vi "M2p_AD_Std.vi"() -> ()   [LabVIEW 2015]
uses:
  spcm_library/spcm_gui_common.llb/element_mode.ctl
  spcm_library/spcm_gui_m2p.llb/element_m2p_ai_channel.ctl
  spcm_library/spcm_gui_m2p.llb/element_m2p_ai_trigger.ctl
  spcm_library/spcm_gui_m2p.llb/element_m2p_clock.ctl
  spcm_library/spcm_gui_common.llb/element_device.ctl
  spcm_library/spcm_gui_common.llb/element_device_infos.ctl
  spcm_library/spcm_gui_m2p.llb/element_m2p_ai_multi_purpose_io.ctl
panel:
  in  "Multi Purpose IO Lines":T1={"X0 Mode"=0, "X1 Mode"=0, "X2 Mode"=0, "X3 Mode"=0, "X0 ASync Send Pulse"=FALSE, "X1 ASync Send Pulse"=FALSE, "X2 ASync Send Pulse"=FALSE, "X3 ASync Send Pulse"=FALSE, "X1 Trigger Mode"=0, "X2 Trigger Mode"=0, "X3 Trigger Mode"=0, "X1 Pulsewidth"=0, "X2 Pulsewidth"=0, "X3 Pulsewidth"=0, "ASync Read Button"=FALSE, "ASync Read"=0, "AI"=TRUE} {"X3 Mode" items=["Disable", "Asynchronous Out", "Asynchronous In", "Trigger Out", "Trigger In", "Clock Out", "Digital In", "Show Run State", "Show Arm State", "Show Sync Arm State"]; "X2 Mode" items=["Disable", "Asynchronous Out", "Asynchronous In", "Trigger Out", "Trigger In", "Clock Out", "Digital In", "Show Run State", "Show Arm State", "Show Sync Arm State"]; "X3 Trigger Mode" items=["Pos. Edge", "Neg. Edge", "Any Edge", "High Level", "Low Level", "PW Long Pos.", "PW Long Neg.", "PW Short Pos.", "PW Short Neg."]; "X2 Trigger Mode" items=["Pos. Edge", "Neg. Edge", "Any Edge", "High Level", "Low Level", "PW Long Pos.", "PW Long Neg.", "PW Short Pos.", "PW Short Neg."]; "X1 Trigger Mode" items=["Pos. Edge", "Neg. Edge", "Any Edge", "High Level", "Low Level", "PW Long Pos.", "PW Long Neg.", "PW Short Pos.", "PW Short Neg."]; "X1 Mode" items=["Disable", "Asynchronous Out", "Asynchronous In", "Trigger Out", "Trigger In", "Clock Out", "Digital In", "Show Run State", "Show Arm State", "Show Sync Arm State"]; "X0 Mode" items=["Disable", "Asynchronous Out", "Trigger Out", "Clock Out", "Show Run State", "Show Arm State", "Show Sync Arm State"]}
  out "Device Infos":T2={"Device Name"="M4i.4451-Exp", "Serial Number"=1122.0, "Mem (MB)"=4096.0}
  in  "Device":T3 {"Device" items=["Card", "digitizerNETBOX"]}
  in  "Clock Settings":T4={"Clock Mode"=0, "Sampling Rate (kHz)"=10000.0, "Clock Output"=FALSE, "Termination"=FALSE, "Ref. Clock (MHz)"=10.0, "Threshold (mV)"=1500} {"Threshold (mV)" min=-5000 max=5000; "Clock Mode" items=["Internal Clock Quartz", "External Clock", "External Reference Clock"]; "Ref. Clock (MHz)" min=0.0 max=125000.0; "Sampling Rate (kHz)" min=1.0 max=5000000.0}
  in  "Trigger Settings":T5={"Trigger Source"=0, "External Trigger"=0, "Level 0 Ext"=1500, "Ext Trig Term"=FALSE, "Channel Trigger"=0, "Level 0 Ch"=0, "Level 1 Ch"=0, "Trigger Delay (Samples)"=0} {"Channel Trigger" items=["None", "Pos. Edge", "Neg. Edge", "Any Edge", "Pos. Rearm", "Neg. Rearm", "Enter Window", "Leave Window", "In Win", "Out Win"]; "External Trigger" items=["None", "Pos. Edge", "Neg. Edge", "Any Edge", "High Level", "Low Level"]; "Trigger Source" items=["Software Trigger", "External Trigger", "Channel 0 Trigger", "Channel 1 Trigger", "Channel 2 Trigger", "Channel 3 Trigger", "Channel 4 Trigger", "Channel 5 Trigger", "Channel 6 Trigger", "Channel 7 Trigger"]; "Trigger Delay (Samples)" max=65535 step=1}
  in  "Quit Button":bool
  in  "AI Channel 7":T6={"Enable"=TRUE, "Input Range "=2, "Termination"=0, "Input Type"=0, "Offset"=0} {"Input Type" items=["Single-ended", "Differential"]; "Termination" items=["1 MOhm", "50 Ohm"]; "Input Range" items=["±200 mV", "±500 mV", "±1000 mV", "±2000 mV", "±5000 mV", "±10000 mV"]}
  in  "AI Channel 6":T6={"Enable"=TRUE, "Input Range "=2, "Termination"=0, "Input Type"=0, "Offset"=0} {"Input Type" items=["Single-ended", "Differential"]; "Termination" items=["1 MOhm", "50 Ohm"]; "Input Range" items=["±200 mV", "±500 mV", "±1000 mV", "±2000 mV", "±5000 mV", "±10000 mV"]}
  in  "AI Channel 5":T6={"Enable"=TRUE, "Input Range "=2, "Termination"=0, "Input Type"=0, "Offset"=0} {"Input Type" items=["Single-ended", "Differential"]; "Termination" items=["1 MOhm", "50 Ohm"]; "Input Range" items=["±200 mV", "±500 mV", "±1000 mV", "±2000 mV", "±5000 mV", "±10000 mV"]}
  in  "AI Channel 4":T6={"Enable"=TRUE, "Input Range "=2, "Termination"=0, "Input Type"=0, "Offset"=0} {"Input Type" items=["Single-ended", "Differential"]; "Termination" items=["1 MOhm", "50 Ohm"]; "Input Range" items=["±200 mV", "±500 mV", "±1000 mV", "±2000 mV", "±5000 mV", "±10000 mV"]}
  in  "AI Channel 3":T6={"Enable"=TRUE, "Input Range "=2, "Termination"=0, "Input Type"=0, "Offset"=0} {"Input Type" items=["Single-ended", "Differential"]; "Termination" items=["1 MOhm", "50 Ohm"]; "Input Range" items=["±200 mV", "±500 mV", "±1000 mV", "±2000 mV", "±5000 mV", "±10000 mV"]}
  in  "AI Channel 2":T6={"Enable"=TRUE, "Input Range "=2, "Termination"=0, "Input Type"=0, "Offset"=0} {"Input Type" items=["Single-ended", "Differential"]; "Termination" items=["1 MOhm", "50 Ohm"]; "Input Range" items=["±200 mV", "±500 mV", "±1000 mV", "±2000 mV", "±5000 mV", "±10000 mV"]}
  in  "AI Channel 1":T6={"Enable"=TRUE, "Input Range "=2, "Termination"=0, "Input Type"=0, "Offset"=0} {"Input Type" items=["Single-ended", "Differential"]; "Termination" items=["1 MOhm", "50 Ohm"]; "Input Range" items=["±200 mV", "±500 mV", "±1000 mV", "±2000 mV", "±5000 mV", "±10000 mV"]}
  in  "AI Channel 0":T6={"Enable"=TRUE, "Input Range "=2, "Termination"=0, "Input Type"=0, "Offset"=0} {"Input Type" items=["Single-ended", "Differential"]; "Termination" items=["1 MOhm", "50 Ohm"]; "Input Range" items=["±200 mV", "±500 mV", "±1000 mV", "±2000 mV", "±5000 mV", "±10000 mV"]}
  in  "Loop Button":bool
  in  "Singleshot Button":bool
  out "Write Setup":bool
  out "Status":string
  in  "Force Trigger Button":bool
  in  "Stop Button":bool
  out "Display Data":sgl[][](graph)
  in  "Mode Setup":T7={"Mode"=0, "Mem"=16384, "Seg"=1024, "Post"=8192, "Pre"=32, "ABA"=16} {"Mode" items=["Singleshot", "Multiple Recording", "Gated Sampling", "ABA Mode"]; "ABA" min=2 max=65535 step=1; "Post" min=4 step=4; "Mem" min=8 step=4; "Pre" min=4 max=8176 step=4; "Seg" min=8 step=4}
  # "M2p AD Standard Example"
  # "Range"
  # "Term"
  # "Type"
  # "Offset"
  # "Mode Settings"
  # "Trigger Settings"
  # "Ch0"
  # "Ch1"
  # "Ch2"
  # "Clock Settings"
  # "Ch3"
  # "Ch4"
  # "Ch5"
  # "Ch6"
  # "Multi Purpose IO"
  # "Ch7"
  # "Mode"
  # "ASync Write"
  # "Trig-Mode"
  # "Trig-Pulsewidth"
  # "ASync Read"
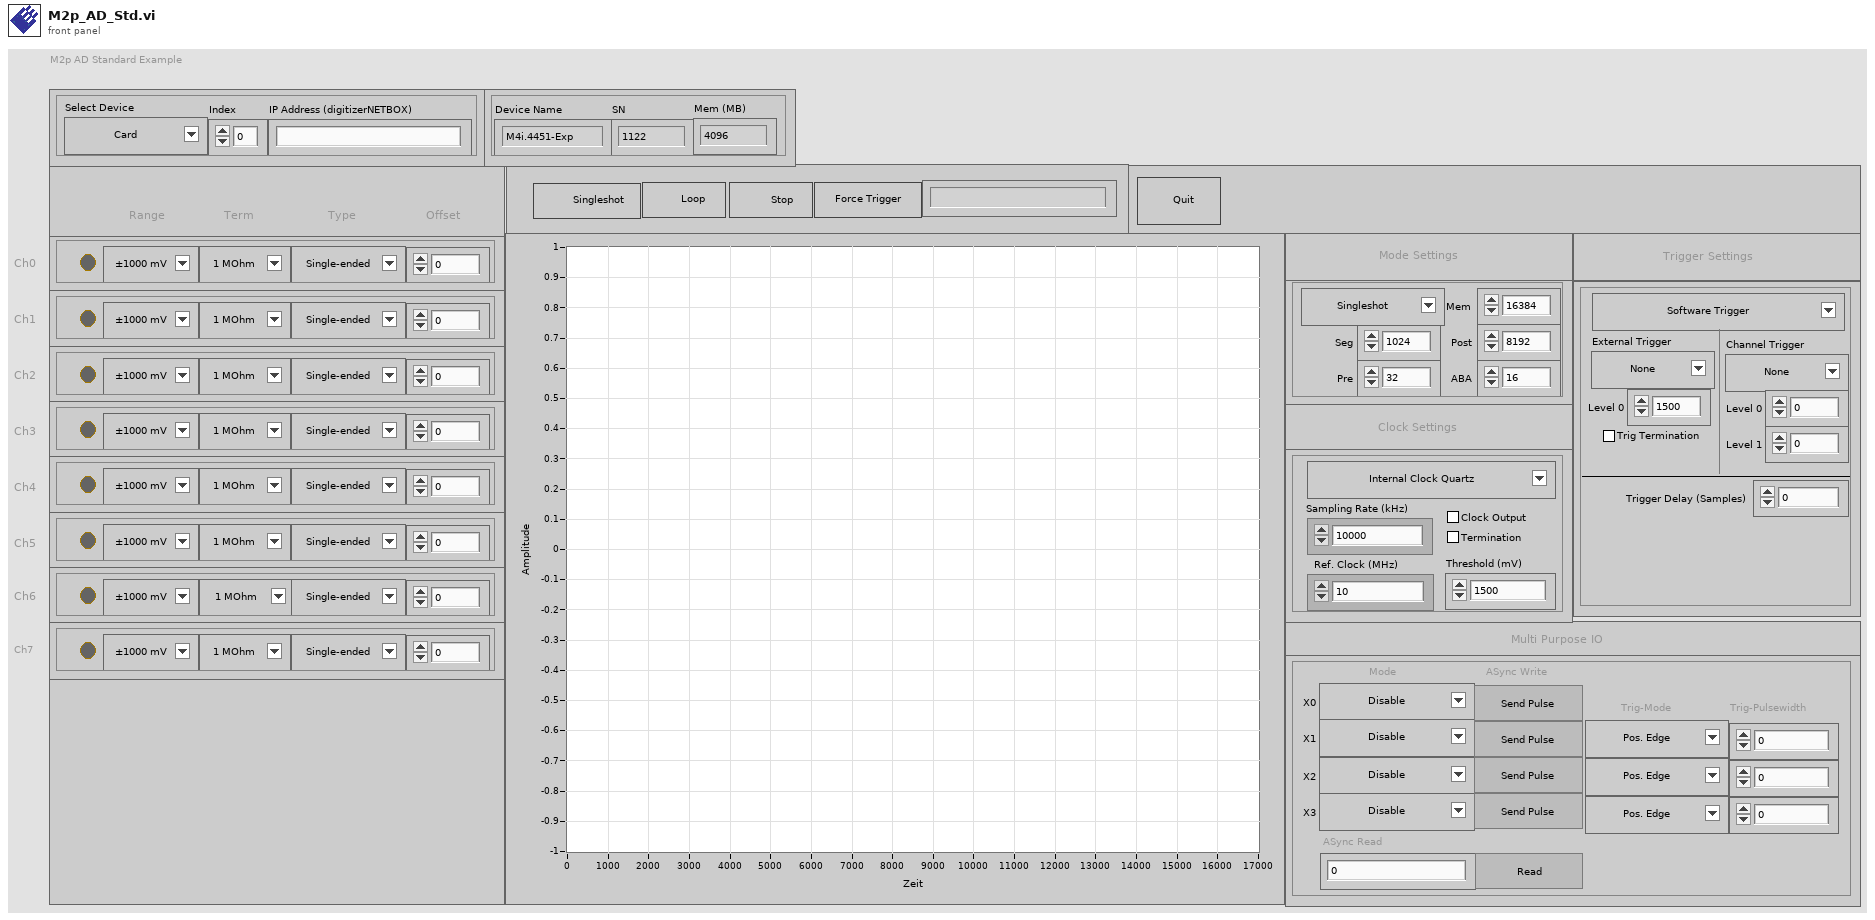
[diagram p1: front panel]
types:
  T1 = typedef "element_m2p_ai_multi_purpose_io.ctl" = cluster{"X0 Mode":u16, "X1 Mode":u16, "X2 Mode":u16, "X3 Mode":u16, "X0 ASync Send Pulse":bool, "X1 ASync Send Pulse":bool, "X2 ASync Send Pulse":bool, "X3 ASync Send Pulse":bool, "X1 Trigger Mode":u16, "X2 Trigger Mode":u16, "X3 Trigger Mode":u16, "X1 Pulsewidth":u32, "X2 Pulsewidth":u32, "X3 Pulsewidth":u32, "ASync Read Button":bool, "ASync Read":i32, "AI":bool}
  T2 = typedef "element_device_infos.ctl" = cluster{"Device Name":string, "Serial Number":dbl, "Mem (MB)":dbl}
  T3 = typedef "element_device.ctl" = cluster{"Index":dbl, "IP Address":string, "Device":u16}
  T4 = typedef "element_m2p_clock.ctl" = cluster{"Clock Mode":u16, "Sampling Rate (kHz)":dbl, "Clock Output":bool, "Termination":bool, "Ref. Clock (MHz)":dbl, "Threshold (mV)":i32}
  T5 = typedef "element_m2p_ai_trigger.ctl" = cluster{"Trigger Source":u16, "External Trigger":u16, "Level 0 Ext":i32, "Ext Trig Term":bool, "Channel Trigger":u16, "Level 0 Ch":i32, "Level 1 Ch":i32, "Trigger Delay (Samples)":u32}
  T6 = typedef "element_m2p_ai_channel.ctl" = cluster{"Enable":bool, "Input Range ":u16, "Termination":u16, "Input Type":u16, "Offset":i32}
  T7 = typedef "element_mode.ctl" = cluster{"Mode":u16, "Mem":u32, "Seg":u32, "Post":u32, "Pre":u32, "ABA":u32}
  T8 = enum16{"Idle", "Init", "Write Setup", "Start", "Acquire", "Read Data", "Stop", "Quit"}
  T9 = cluster{"Card Type":i32, "Inst Mem (high part)":i32, "Inst Mem (low part)":i32, "Serial Number":i32, "Function Type":i32, "Installed Features":i32, "Base Card Version":i32, "Module Version":i32, "Extension Version":i32, "Production Date":i32, "Max Sampling Rate":i32, "Max Channels":i32, "Demo Card":i32}
  T10 = cluster{"Card Name":string, "SN":i32, "Mem (MB)":i32}
  T11 = cluster{"AI Channels":i32, "AI Ranges":i32, "Input Ranges (mV)":i32[], "Programmable Offset":i32, "Termination Available":bool, "SE/Diff switchable":bool, "Offset in per cent/mV":bool, "Offset Calibration":bool, "Gain Calibration":bool, "Offset with open inputs":bool, "AI Range Strings[]":string[], "Bit Resolution":i32, "AC Coupling available":bool, "BW Limit available":bool, "AI Path count":i32}
  T12 = enum16{"Idle", "Init", "Write Setup", "Start", "Acquire", "Read Data", "Quit"}
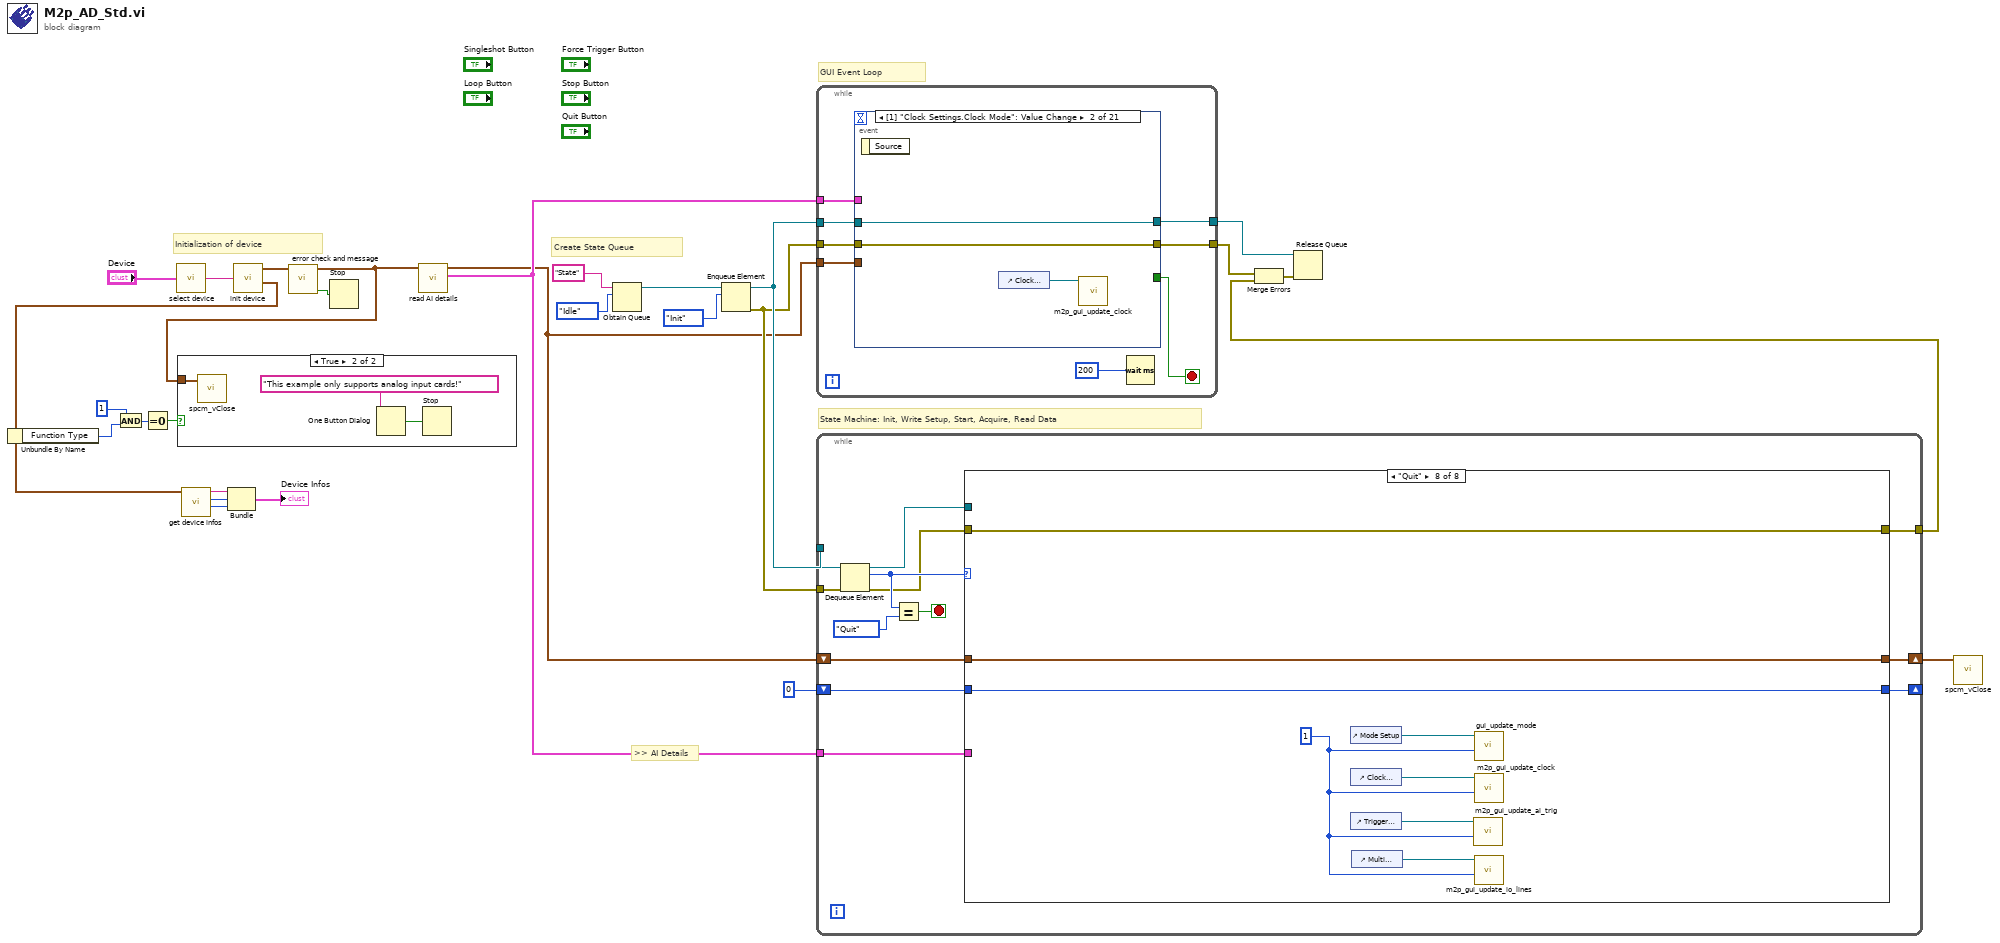
[diagram p0: block diagram]
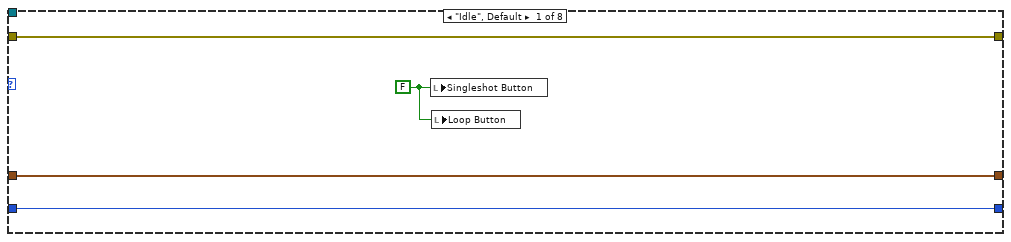
[diagram p3: hidden frame]
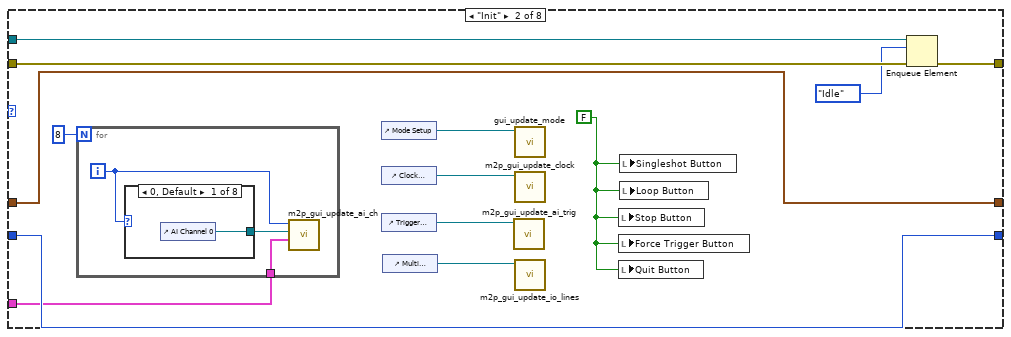
[diagram p4: hidden frame]
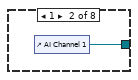
[diagram p5: hidden frame]
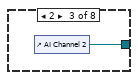
[diagram p6: hidden frame]
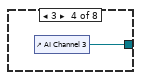
[diagram p7: hidden frame]
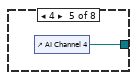
[diagram p8: hidden frame]
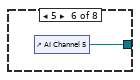
[diagram p9: hidden frame]
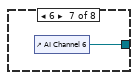
[diagram p10: hidden frame]
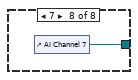
[diagram p11: hidden frame]
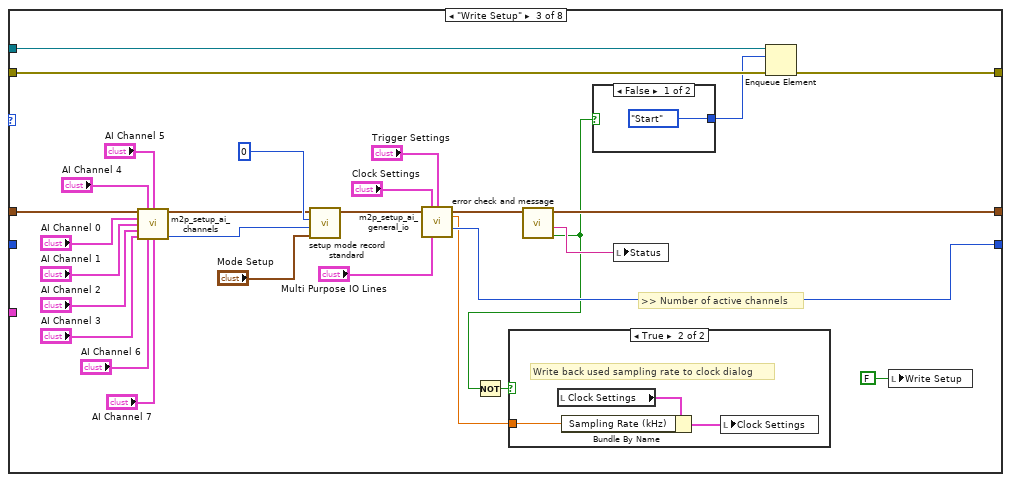
[diagram p12: hidden frame]
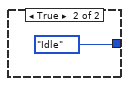
[diagram p14: hidden frame]
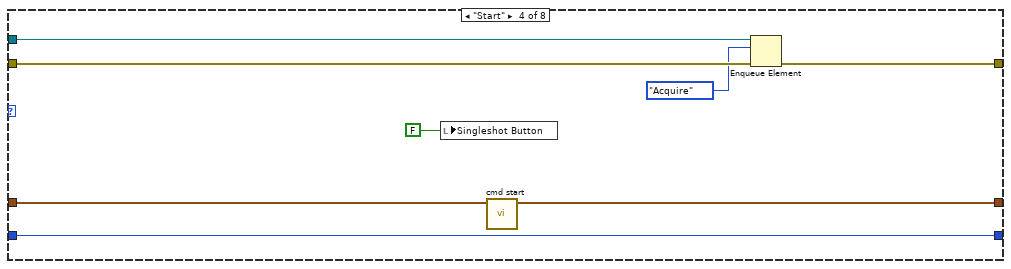
[diagram p15: hidden frame]
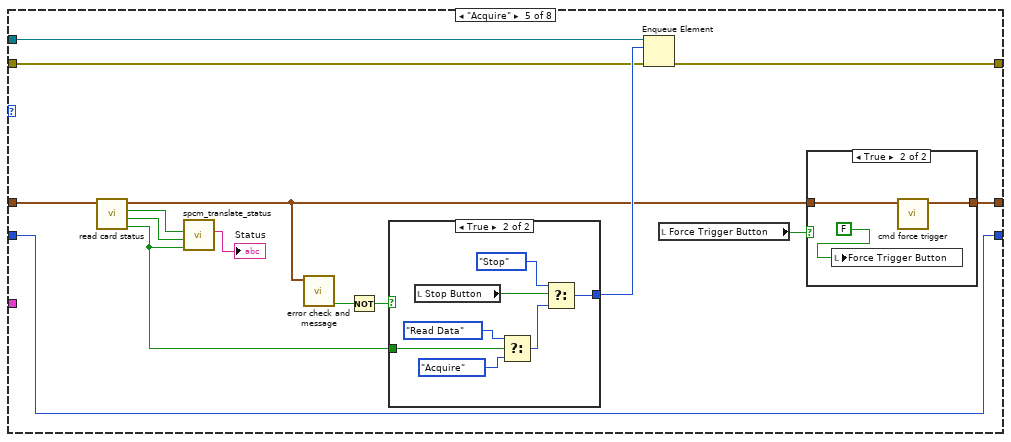
[diagram p16: hidden frame]
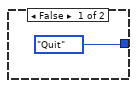
[diagram p17: hidden frame]
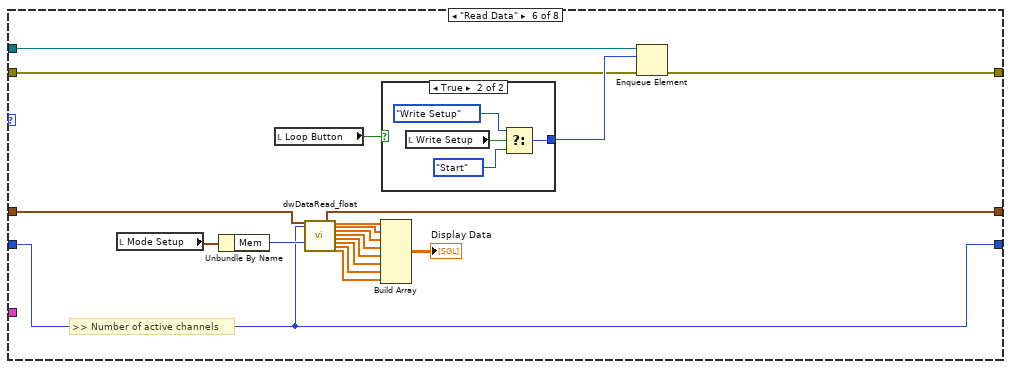
[diagram p19: hidden frame]
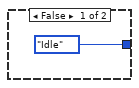
[diagram p20: hidden frame]
diagram:
  # ">> AI Details"
  # "Initialization of device"
  # "Create State Queue"
  # "State Machine: Init, Write Setup, Start, Acquire, Read Data"
  # "GUI Event Loop"
  n1 = call "select device.vi"("Device"="Device") -> ("device string"=w28:string)  [unwired: 4 in]
  n2 = call "init device.vi"("Device String"=w28) -> ("Card Info Out"=w27:cluster{"Card Handle":u64, "Error Code":u32}, "Card Information"=w13:T9)  [unwired: 4 in]
  n3 = Unbundle By Name(w13) -> ("Function Type"=w17:i32)
  n4 = And(x=1, y=w17) -> (x .and. y?=w16:i32)
  n5 = Equal To 0?(x=w16) -> (x = 0?=w14:bool)
  n6 = call "get device infos.vi"("Card Information"=w13) -> ("Mem (MB)"=w20:i32, "SN"=w19:i32, "Card Name"=w18:string)  [unwired: 8 in]
  n7 = Bundle("Card Name"=w18, "SN"=w19, "Mem (MB)"=w20) -> (→"Device Infos":T10)  [unwired: 1 in]
  n8 = call "error check and message.vi"("Card Info In"=w27) -> ("Error occurred"=w26:bool, "Card Info Out"=w5:cluster{"Card Handle":u64, "Error Code":u32})  [unwired: 4 in, 1 out]
  n9 = case shown="True" w14 {
    tunnel: w5 -> [_ w29]
    frame False {
    }
    frame True {
      n10 = call "spcm_vClose.vi"("Card Info In"=w29) -> ()  [unwired: 7 in]
      n11 = One Button Dialog(message="This example only supports analog input cards!") -> (true=w30:bool)  [unwired: 1 in]
      n12 = Stop(stop? (T)=w30) -> ()
    }
  }
  n13 = Stop(stop? (T)=w26) -> ()
  n14 = call "read AI details.vi"("Card Info In"=w5) -> ("AI Details"=w4:T11, "Card Info Out"=w3:cluster{"Card Handle":u64, "Error Code":u32})  [unwired: 5 in]
  n15 = Obtain Queue(name (unnamed)="State", element data type=T8."Idle") -> (queue out=w23:refnum<queue>)  [unwired: 3 in, 2 out]
  n16 = Enqueue Element(queue=w23, element=T8."Init") -> (queue out=w24:refnum<queue>, error out=w8:errorcluster)  [unwired: 2 in, 1 out]
  n17 = while {
    tunnel: w24 -> [w37]
    tunnel: [w38] -> w9
    tunnel: [w34] -> w12
    tunnel: w8 -> [w35]
    tunnel: w4 -> [w33]
    tunnel: w3 -> [w32]
    stop <- w36 stop-if-true
    n18 = event shown="[1] \"Clock Settings.Clock Mode\": Value Change" {
      selector: _ -> [_ _ _ _ _ _ _ _ _ _ _ _ _ _ _ _ _ _ _ _ _]
      dyn-events: _ -> [_ _ _ _ _ _ _ _ _ _ _ _ _ _ _ _ _ _ _ _ _]
      timeout: _ -> [_ _ _ _ _ _ _ _ _ _ _ _ _ _ _ _ _ _ _ _ _]
      tunnel: [_ _ _ _ _ _ _ _ _ _ _ _ _ _ _ _ _ _ _ TRUE _] -> w36
      tunnel: [w41 w45 w48 w50 w58 w63 w68 w73 w79 w84 w89 w94 w99 w104 w109 w114 w119 w124 w129 w134 w138] -> w38
      tunnel: w37 -> [w41 w45 w48 w50 w58 w63 w68 w73 w79 w84 w89 w94 w99 w104 w109 w114 w119 w123 w128 w135 w138]
      tunnel: [w40 w44 w47 w51 w57 w62 w67 w72 w78 w83 w88 w93 w98 w103 w108 w113 w118 w121 w126 w132 w137] -> w34
      tunnel: w35 -> [w40 w44 w47 w51 w57 w62 w67 w72 w78 w83 w88 w93 w98 w103 w108 w113 w118 w122 w127 w131 w137]
      tunnel: w33 -> [_ _ _ _ _ _ _ _ _ w80 w86 w91 w96 w101 w106 w111 w116 _ _ _ _]
      tunnel: w32 -> [_ _ _ w53 w55 w60 w65 w70 w77 _ _ _ _ _ _ _ _ _ _ _ _]
      event Value Change {
        n19 = event-data ("Ereignisdatenknoten")() -> ()  [unwired: 1 in, 1 out]
        n20 = control-ref of="Mode Setup"() -> (w42:refnum<vi>)
        n21 = call "gui_update_mode.vi"("Referenz Mode Settings"=w42) -> ()  [unwired: 11 in]
      }
      event Value Change {
        n22 = event-data() -> ()  [unwired: 1 in, 1 out]
        n23 = control-ref of="Clock Settings"() -> (w43:refnum<vi>)
        n24 = call "m2p_gui_update_clock.vi"("Cluster Reference"=w43) -> ()  [unwired: 11 in]
      }
      event Value Change {
        n25 = event-data() -> ()  [unwired: 1 in, 1 out]
        n26 = control-ref of="Trigger Settings"() -> (w46:refnum<vi>)
        n27 = call "m2p_gui_update_ai_trig.vi"("Trigger Settings Reference"=w46) -> ()  [unwired: 10 in]
      }
      event Value Change {
        n28 = event-data() -> ()  [unwired: 1 in, 1 out]
        n29 = local read "Multi Purpose IO Lines"() -> (w52:T1)
        n30 = control-ref of="Multi Purpose IO Lines"() -> (w49:refnum<vi>)
        n31 = call "m2p_gui_update_io_lines.vi"("Cluster Reference"=w49) -> ()  [unwired: 11 in]
        n32 = call "setup M2p IO lines.vi"("Multi Purpose IO Lines"=w52, "Card Info In"=w53) -> ()  [unwired: 1 in, 1 out]
      }
      event Value Change {
        n33 = event-data() -> ()  [unwired: 1 in, 1 out]
        n34 = call "write M2p async io.vi"("Card Info In"=w55, "XIO Index"=0) -> ()  [unwired: 4 in, 1 out]
        n35 = One Button Dialog(message="X0: Send Pulse") -> ()  [unwired: 1 in, 1 out]
      }
      event Value Change {
        n36 = event-data() -> ()  [unwired: 1 in, 1 out]
        n37 = call "write M2p async io.vi"("Card Info In"=w60, "XIO Index"=1) -> ()  [unwired: 4 in, 1 out]
        n38 = One Button Dialog(message="X1: Send Pulse") -> ()  [unwired: 1 in, 1 out]
      }
      event Value Change {
        n39 = event-data() -> ()  [unwired: 1 in, 1 out]
        n40 = call "write M2p async io.vi"("Card Info In"=w65, "XIO Index"=2) -> ()  [unwired: 4 in, 1 out]
        n41 = One Button Dialog(message="X2: Send Pulse") -> ()  [unwired: 1 in, 1 out]
      }
      event Value Change {
        n42 = event-data() -> ()  [unwired: 1 in, 1 out]
        n43 = call "write M2p async io.vi"("Card Info In"=w70, "XIO Index"=3) -> ()  [unwired: 4 in, 1 out]
        n44 = One Button Dialog(message="X3: Send Pulse") -> ()  [unwired: 1 in, 1 out]
      }
      event Value Change {
        n45 = event-data() -> ()  [unwired: 1 in, 1 out]
        n46 = call "read M2p async io.vi"("Card Info In"=w77) -> ("ASync Read"=w76:i32)  [unwired: 5 in, 1 out]
        n47 = local read "Multi Purpose IO Lines"() -> (w75:T1)
        n48 = Bundle By Name(cluster=w75, "ASync Read"=w76) -> (w74:T1)
        n49 = local write "Multi Purpose IO Lines"(w74) -> ()
      }
      event Value Change {
        n50 = event-data() -> ()  [unwired: 1 in, 1 out]
        n51 = control-ref of="AI Channel 0"() -> (w81:refnum<vi>)
        n52 = call "m2p_gui_update_ai_ch.vi"("AI Details"=w80, "Cluster Referenz"=w81, "Channel Index"=0) -> ()  [unwired: 9 in]
      }
      event Value Change {
        n53 = event-data() -> ()  [unwired: 1 in, 1 out]
        n54 = control-ref of="AI Channel 1"() -> (w85:refnum<vi>)
        n55 = call "m2p_gui_update_ai_ch.vi"("AI Details"=w86, "Cluster Referenz"=w85, "Channel Index"=1) -> ()  [unwired: 9 in]
      }
      event Value Change {
        n56 = event-data() -> ()  [unwired: 1 in, 1 out]
        n57 = control-ref of="AI Channel 2"() -> (w90:refnum<vi>)
        n58 = call "m2p_gui_update_ai_ch.vi"("AI Details"=w91, "Cluster Referenz"=w90, "Channel Index"=2) -> ()  [unwired: 9 in]
      }
      event Value Change {
        n59 = event-data() -> ()  [unwired: 1 in, 1 out]
        n60 = control-ref of="AI Channel 3"() -> (w95:refnum<vi>)
        n61 = call "m2p_gui_update_ai_ch.vi"("AI Details"=w96, "Cluster Referenz"=w95, "Channel Index"=3) -> ()  [unwired: 9 in]
      }
      event Value Change {
        n62 = event-data() -> ()  [unwired: 1 in, 1 out]
        n63 = control-ref of="AI Channel 4"() -> (w100:refnum<vi>)
        n64 = call "m2p_gui_update_ai_ch.vi"("AI Details"=w101, "Cluster Referenz"=w100, "Channel Index"=4) -> ()  [unwired: 9 in]
      }
      event Value Change {
        n65 = event-data() -> ()  [unwired: 1 in, 1 out]
        n66 = control-ref of="AI Channel 5"() -> (w105:refnum<vi>)
        n67 = call "m2p_gui_update_ai_ch.vi"("AI Details"=w106, "Cluster Referenz"=w105, "Channel Index"=5) -> ()  [unwired: 9 in]
      }
      event Value Change {
        n68 = event-data() -> ()  [unwired: 1 in, 1 out]
        n69 = control-ref of="AI Channel 6"() -> (w110:refnum<vi>)
        n70 = call "m2p_gui_update_ai_ch.vi"("AI Details"=w111, "Cluster Referenz"=w110, "Channel Index"=6) -> ()  [unwired: 9 in]
      }
      event Value Change {
        n71 = event-data() -> ()  [unwired: 1 in, 1 out]
        n72 = control-ref of="AI Channel 7"() -> (w115:refnum<vi>)
        n73 = call "m2p_gui_update_ai_ch.vi"("AI Details"=w116, "Cluster Referenz"=w115, "Channel Index"=7) -> ()  [unwired: 9 in]
      }
      event "Singleshot Button", "Loop Button": Value Change {
        n74 = event-data() -> ()  [unwired: 1 in, 1 out]
        n75 = Enqueue Element(queue=w123, element=T8."Write Setup", error in (no error)=w122) -> (queue out=w124:refnum<queue>, error out=w121:errorcluster)  [unwired: 1 in, 1 out]
      }
      event "Stop Button": Value Change {
        n76 = event-data() -> ()  [unwired: 1 in, 1 out]
        n77 = Enqueue Element(queue=w128, element=T8."Idle", error in (no error)=w127) -> (queue out=w129:refnum<queue>, error out=w126:errorcluster)  [unwired: 1 in, 1 out]
      }
      event "Quit Button": Value Change {
        n78 = event-data() -> ()  [unwired: 1 in, 1 out]
        n79 = Enqueue Element(queue=w135, element=T8."Quit", error in (no error)=w131) -> (queue out=w134:refnum<queue>, error out=w132:errorcluster)  [unwired: 1 in, 1 out]
      }
      event Value Change {
        n80 = event-data() -> ()  [unwired: 1 in, 1 out]
        "Write Setup" <- TRUE
      }
    }
    n81 = Wait (ms)(milliseconds to wait=200) -> ()  [unwired: 1 out]
  }
  n82 = while {
    tunnel: w24 -> [w151]
    shift-right: [w149] -> w22
    shift-left: w3 -> [w150]
    shift-right: [w144] -> _
    shift-left: 0 -> [w145]
    tunnel: [w143] -> w11
    tunnel: w8 -> [w142]
    tunnel: w4 -> [w139]
    stop <- w147 stop-if-true
    n83 = Dequeue Element(queue=w151, error in (no error)=w142) -> (queue out=w146:refnum<queue>, element=w148:T8, error out=w141:errorcluster)  [unwired: 1 in, 1 out]
    n84 = Equal?(x=w148, y=T8."Quit") -> (x = y?=w147:bool)
    n85 = case shown="\"Quit\"" w148 {
      tunnel: w150 -> [w155 w163 w195 w220 w226 w258 w276 w287]
      tunnel: [w155 w163 w205 w219 w233 w263 w275 w287] -> w149
      tunnel: w146 -> [_ w167 w208 w217 w230 w260 w280 _]
      tunnel: w145 -> [w154 w162 _ w221 w229 w257 w274 w286]
      tunnel: [w154 w162 w198 w221 w229 w257 w274 w286] -> w144
      tunnel: [w153 w166 w206 w216 w228 w255 w278 w288] -> w143
      tunnel: w141 -> [w153 w165 w207 w218 w227 w254 w279 w288]
      tunnel: w139 -> [_ w159 _ _ _ _ _ _]
      frame "Idle", Default {
        w152 = FALSE
        n86 = local write "Singleshot Button"(w152) -> ()
        n87 = local write "Loop Button"(w152) -> ()
      }
      frame "Init" {
        w161 = FALSE
        n88 = for {
          N: 8 -> [_]
          tunnel: w159 -> [w169]
          i -> [w171]
          n89 = case shown="0, Default" w171 {
            tunnel: [w172 w173 w174 w175 w176 w177 w178 w179] -> w170
            frame 0, Default {
              n90 = control-ref of="AI Channel 0"() -> (w172:refnum<vi>)
            }
            frame 1 {
              n91 = control-ref of="AI Channel 1"() -> (w173:refnum<vi>)
            }
            frame 2 {
              n92 = control-ref of="AI Channel 2"() -> (w174:refnum<vi>)
            }
            frame 3 {
              n93 = control-ref of="AI Channel 3"() -> (w175:refnum<vi>)
            }
            frame 4 {
              n94 = control-ref of="AI Channel 4"() -> (w176:refnum<vi>)
            }
            frame 5 {
              n95 = control-ref of="AI Channel 5"() -> (w177:refnum<vi>)
            }
            frame 6 {
              n96 = control-ref of="AI Channel 6"() -> (w178:refnum<vi>)
            }
            frame 7 {
              n97 = control-ref of="AI Channel 7"() -> (w179:refnum<vi>)
            }
          }
          n98 = call "m2p_gui_update_ai_ch.vi"("AI Details"=w169, "Cluster Referenz"=w170, "Channel Index"=w171) -> ()  [unwired: 9 in]
        }
        n99 = control-ref of="Mode Setup"() -> (w168:refnum<vi>)
        n100 = control-ref of="Clock Settings"() -> (w158:refnum<vi>)
        n101 = control-ref of="Trigger Settings"() -> (w156:refnum<vi>)
        n102 = control-ref of="Multi Purpose IO Lines"() -> (w157:refnum<vi>)
        n103 = call "m2p_gui_update_ai_trig.vi"("Trigger Settings Reference"=w156) -> ()  [unwired: 10 in]
        n104 = call "gui_update_mode.vi"("Referenz Mode Settings"=w168) -> ()  [unwired: 11 in]
        n105 = call "m2p_gui_update_clock.vi"("Cluster Reference"=w158) -> ()  [unwired: 11 in]
        n106 = call "m2p_gui_update_io_lines.vi"("Cluster Reference"=w157) -> ()  [unwired: 11 in]
        n107 = local write "Stop Button"(w161) -> ()
        n108 = local write "Force Trigger Button"(w161) -> ()
        n109 = local write "Quit Button"(w161) -> ()
        n110 = local write "Singleshot Button"(w161) -> ()
        n111 = local write "Loop Button"(w161) -> ()
        n112 = Enqueue Element(queue=w167, element=T8."Idle", error in (no error)=w165) -> (error out=w166:errorcluster)  [unwired: 1 in, 2 out]
      }
      frame "Write Setup" {
        # ">> Number of active channels"
        n113 = call "m2p_setup_ai_channels.vi"("Card Info In"=w195, "AI Channel 4"="AI Channel 4", "AI Channel 5"="AI Channel 5", "AI Channel 0"="AI Channel 0", "AI Channel 1"="AI Channel 1", "AI Channel 2"="AI Channel 2", "AI Channel 3"="AI Channel 3", "AI Channel 6"="AI Channel 6", "AI Channel 7"="AI Channel 7") -> ("Card Info Out"=w194:cluster{"Card Handle":u64, "Error Code":u32}, "ChMask"=w186:i32)  [unwired: 5 in]
        n114 = call "setup mode record standard.vi"("Mode Setup"="Mode Setup", "Channel Mask Low"=w186, "Channel Mask High"=0, "Card Info In"=w194) -> ("Card Info Out"=w200:cluster{"Card Handle":u64, "Error Code":u32})  [unwired: 2 in, 1 out]
        n115 = call "m2p_setup_ai_general_io.vi"("Card Info In"=w200, "Clock Settings"="Clock Settings", "Trigger Settings"="Trigger Settings", "Multi Purpose IO Lines"="Multi Purpose IO Lines") -> ("Card Info Out"=w199:cluster{"Card Handle":u64, "Error Code":u32}, "Used Sampling Rate (kS)"=w197:dbl, "Channel Count"=w198:i32)  [unwired: 8 in, 1 out]
        n116 = call "error check and message.vi"("Card Info In"=w199) -> ("Error occurred"=w181:bool, "Error Message"=w203:string, "Card Info Out"=w205:cluster{"Card Handle":u64, "Error Code":u32})  [unwired: 4 in]
        n117 = Not(x=w181) -> (.not. x?=w182:bool)
        n118 = case shown="True" w182 {
          tunnel: w197 -> [_ w211]
          frame False {
          }
          frame True {
            # "Write back used sampling rate to clock dialog"
            n119 = local read "Clock Settings"() -> (w210:T4)
            n120 = Bundle By Name(cluster=w210, "Sampling Rate (kHz)"=w211) -> (w209:T4)
            n121 = local write "Clock Settings"(w209) -> ()
          }
        }
        n122 = case shown="False" w181 {
          tunnel: [T8."Start" T12."Idle"] -> w204
          frame False {
          }
          frame True {
          }
        }
        n123 = local write "Status"(w203) -> ()
        n124 = Enqueue Element(queue=w208, element=w204, error in (no error)=w207) -> (error out=w206:errorcluster)  [unwired: 1 in, 2 out]
        n125 = local write "Write Setup"(FALSE) -> ()
      }
      frame "Start" {
        n126 = local write "Singleshot Button"(FALSE) -> ()
        n127 = call "cmd start.vi"("Card Info In"=w220) -> ("Card Info Out"=w219:cluster{"Card Handle":u64, "Error Code":u32})  [unwired: 6 in]
        n128 = Enqueue Element(queue=w217, element=T8."Acquire", error in (no error)=w218) -> (error out=w216:errorcluster)  [unwired: 1 in, 2 out]
      }
      frame "Acquire" {
        n129 = call "read card status.vi"("Card Info In"=w226) -> ("Card ready"=w232:bool, "Trigger detected"=w235:bool, "Pretrigger full"=w236:bool, "Card Info Out"=w223:cluster{"Card Handle":u64, "Error Code":u32})  [unwired: 3 in]
        n130 = call "spcm_translate_status.vi"("Ready"=w232, "Trigger"=w235, "Pretrigger"=w236) -> ("Text"=→"Status":string)  [unwired: 4 in]
        n131 = call "error check and message.vi"("Card Info In"=w223) -> ("Error occurred"=w224:bool)  [unwired: 4 in, 2 out]
        n132 = Not(x=w224) -> (.not. x?=w225:bool)
        n133 = case shown="True" w225 {
          tunnel: [T12."Quit" w244] -> w234
          tunnel: w232 -> [_ w243]
          frame False {
          }
          frame True {
            n134 = local read "Stop Button"() -> (w238:bool)
            n135 = Select(t=T8."Read Data", s=w243, f=T8."Acquire") -> (s? t:f=w242:T8)
            n136 = Select(t=T8."Stop", s=w238, f=w242) -> (s? t:f=w244:T8)
          }
        }
        n137 = Enqueue Element(queue=w230, element=w234, error in (no error)=w227) -> (error out=w228:errorcluster)  [unwired: 1 in, 2 out]
        n138 = local read "Force Trigger Button"() -> (w222:bool)
        n139 = case shown="True" w222 {
          tunnel: w223 -> [w245 w248]
          tunnel: [w245 w247] -> w233
          frame False {
          }
          frame True {
            n140 = local write "Force Trigger Button"(FALSE) -> ()
            n141 = call "cmd force trigger.vi"("Card Info In"=w248) -> ("Card Info Out"=w247:cluster{"Card Handle":u64, "Error Code":u32})  [unwired: 6 in]
          }
        }
      }
      frame "Read Data" {
        # ">> Number of active channels"
        n142 = local read "Mode Setup"() -> (w264:T7)
        n143 = Unbundle By Name(w264) -> ("Mem"=w259:u32)
        n144 = local read "Loop Button"() -> (w253:bool)
        n145 = call "dwDataRead_float.vi"("Card Info In"=w258, "Channel Count"=w257, "Length (Samples per Channel)"=w259) -> ("Card Info Out"=w263:cluster{"Card Handle":u64, "Error Code":u32}, "Ch 0"=w267:sgl[], "Ch 1"=w266:sgl[], "Ch 2"=w265:sgl[], "Ch 3"=w262:sgl[], "Ch 4"=w252:sgl[], "Ch 5"=w251:sgl[], "Ch 6"=w250:sgl[], "Ch 7"=w249:sgl[])  [unwired: 8 in, 8 out]
        n146 = Build Array(w267, w266, w265, w262, w252, w251, w250, w249) -> (→"Display Data":sgl[][])
        n147 = case shown="True" w253 {
          tunnel: [T12."Idle" w272] -> w256
          frame False {
          }
          frame True {
            n148 = local read "Write Setup"() -> (w269:bool)
            n149 = Select(t=T8."Write Setup", s=w269, f=T8."Start") -> (s? t:f=w272:T8)
          }
        }
        n150 = Enqueue Element(queue=w260, element=w256, error in (no error)=w254) -> (error out=w255:errorcluster)  [unwired: 1 in, 2 out]
      }
      frame "Stop" {
        n151 = call "cmd stop.vi"("Card Info In"=w276) -> ("Card Info Out"=w275:cluster{"Card Handle":u64, "Error Code":u32})  [unwired: 6 in]
        n152 = local write "Status"("Stopped") -> ()
        n153 = Enqueue Element(queue=w280, element=T8."Idle", error in (no error)=w279) -> (error out=w278:errorcluster)  [unwired: 1 in, 2 out]
      }
      frame "Quit" {
        w285 = 1
        n154 = control-ref of="Mode Setup"() -> (w284:refnum<vi>)
        n155 = control-ref of="Clock Settings"() -> (w283:refnum<vi>)
        n156 = control-ref of="Trigger Settings"() -> (w281:refnum<vi>)
        n157 = control-ref of="Multi Purpose IO Lines"() -> (w282:refnum<vi>)
        n158 = call "m2p_gui_update_ai_trig.vi"("Enable Mode"=w285, "Trigger Settings Reference"=w281) -> ()  [unwired: 9 in]
        n159 = call "gui_update_mode.vi"("Enable Mode"=w285, "Referenz Mode Settings"=w284) -> ()  [unwired: 10 in]
        n160 = call "m2p_gui_update_clock.vi"("Enable Mode"=w285, "Cluster Reference"=w283) -> ()  [unwired: 10 in]
        n161 = call "m2p_gui_update_io_lines.vi"("Enable Mode"=w285, "Cluster Reference"=w282) -> ()  [unwired: 10 in]
      }
    }
  }
  n162 = Merge Errors(w12, w11) -> (w10:errorcluster)
  n163 = Release Queue(queue=w9, error in (no error)=w10) -> ()  [unwired: 1 in, 3 out]
  n164 = call "spcm_vClose.vi"("Card Info In"=w22) -> ()  [unwired: 7 in]
